vi "Redraw Tree.vi"(8 "error in (no error)":errorcluster, 11 "Test Executive Builder Model in":refnum<class "Test Executive Builder Model.lvclass">) -> (0 "error out":errorcluster, 3 "Test Executive Builder Model out":refnum<class "Test Executive Builder Model.lvclass">)   [LabVIEW 2017, in "Test Executive Builder Model.lvclass"]
uses:
  Test Executive Builder Model.lvclass
  <vilib>/gpm_packages/@cs/mva-core/Source/IModel/IModel/IModel.lvclass
  C:/Users/jonmc/Documents/Git/Test Executive Builder/gpm_packages/@cs/mva-core/Source/IModel/IModel/IModel.lvclass
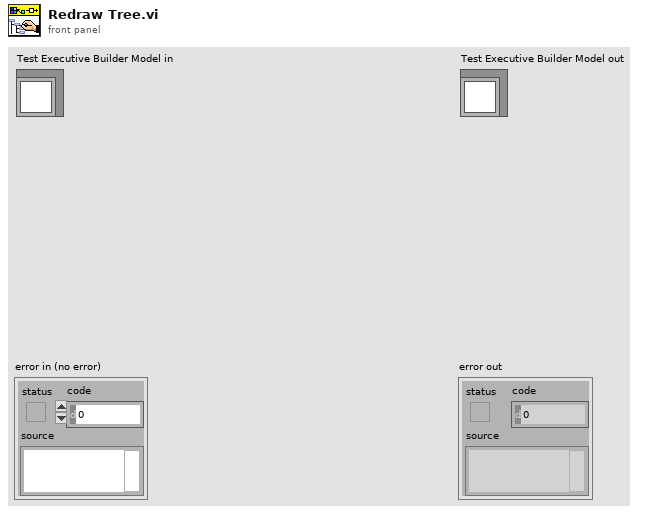
[diagram p1: front panel]
types:
  T1 = cluster{"Left Cell String":string, "Child Text":string[], "Child Tag":string, "Item Indent":i32, "Child Only?":bool, "Glyph Index":i32}[]
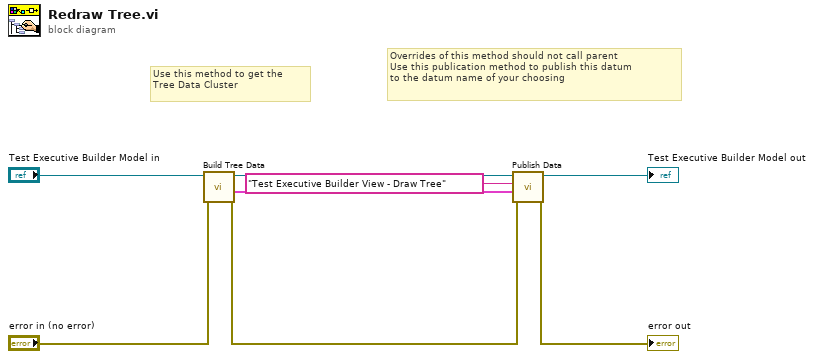
[diagram p0: block diagram]
diagram:
  # "Use this method to get the\nTree Data Cluster"
  # "Overrides of this method should not call parent\nUse this publication method to publish this datum\nto the datum name of your choosing"
  n1 = call "Build Tree Data.vi"("error in (no error)"="error in (no error)", "Test Executive Builder Model in"="Test Executive Builder Model in") -> ("error out"=w2:errorcluster, "Tree Data"=w1:T1, "Test Executive Builder Model out"=w4:refnum<class "Test Executive Builder Model.lvclass">)  [unwired: 7 in]
  n2 = call <vilib>:"Publish Data.vi"("error in (no error)"=w2, "Data to Publish"=w1, "Datum Name"="Test Executive Builder View - Draw Tree", "IModel in"=w4) -> ("error out"=→"error out":errorcluster, "IModel out"=→"Test Executive Builder Model out":refnum<class "Test Executive Builder Model.lvclass">)  [unwired: 6 in]
